vi "Invalid Application Refnum.vi"() -> ()   [LabVIEW 2017, in "Transparent Assertions.Tests.lvlib" / "Assert Refnum.lvlib"]
uses:
  Assert Refnum.lvlib
  src/Transparent Assertions/Transparent Assertions.lvlib
panel:
  out "error out":errorcluster
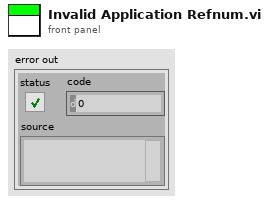
[diagram p1: front panel]
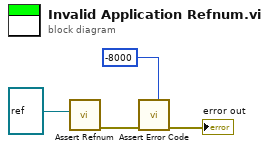
[diagram p0: block diagram]
diagram:
  n1 = call "Assert Refnum.vi"("Refnum"=refnum<vi> refnum ("App Refnum")) -> ("error out"=w4:errorcluster)  [unwired: 10 in]
  n2 = call "Assert Error Code.vi"("Expected"=-8000, "error in (no error)"=w4) -> ("error out"=→"error out":errorcluster)  [unwired: 9 in]
